vi "DSF.Engine.Transceiver Thread.Command.Transfer Group.vi"(8 "error in (no error)":errorcluster, 9 "Command":T1, 10 "Transfer Group":refnum<class "DSF.Engine.Transfer Group.lvclass">, 11 "Transceiver Thread in":refnum<class "DSF.Engine.Transceiver Thread.lvclass">) -> (0 "error out":errorcluster, 3 "Transceiver Thread out":refnum<class "DSF.Engine.Transceiver Thread.lvclass">)   [LabVIEW 2017, in "DSF.Engine.lvlib" / "DSF.Engine.Transceiver Thread.lvclass"]
uses:
  DSF.Engine.Transceiver Thread.lvclass
  Transfer/DSF.Engine.Transfer Group.lvclass
  Interface/DSF.Engine.Interface.Transceiver.Command.ctl
  Interface/DSF.Engine.Interface.Transceiver.Command Data.ctl
  Interface/DSF.Engine.Interface.Transceiver.Command Parameters.ctl
  DSF.Engine.Transceiver Thread.lvclass/DSF.Engine.Transceiver Thread.ctl
  Transfer/DSF.Engine.Transfer Group.lvclass/DSF.Engine.Transfer Group.ctl
  Timing/DSF.Engine.Timing.lvclass/DSF.Engine.Timing.ctl
  Interface/DSF.Engine.Interface.Transceiver.Write.Command.vi
  Interface/DSF.Engine.Interface.Transceiver.lvclass
  Timing/DSF.Engine.Timing.lvclass
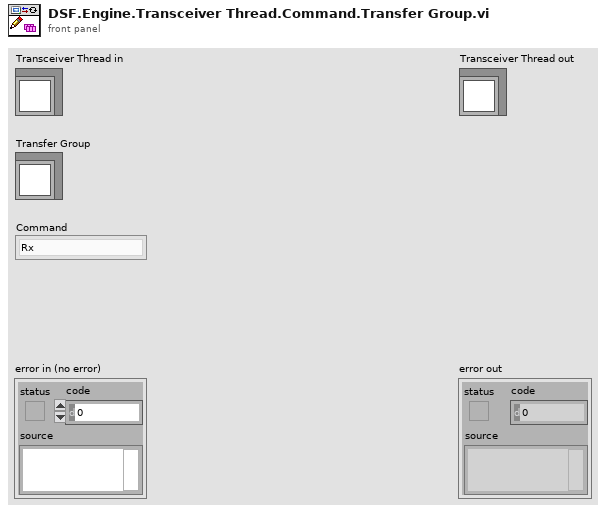
[diagram p1: front panel]
types:
  T1 = typedef "DSF.Engine.lvlib/DSF.Engine.Interface.Transceiver.lvclass/DSF.Engine.Interface.Transceiver.Command.ctl" = enum8{"Rx", "Tx", "Shutdown"}
  T2 = cluster{"Transfer Group ID":i32, "unused":i32, "Transfer Group iteration":u64}
  T3 = typedef "DSF.Engine.lvlib/DSF.Engine.Interface.Transceiver.lvclass/DSF.Engine.Interface.Transceiver.Command Parameters.ctl" = cluster{"arg1":u64, "arg2":u64}
  T4 = typedef "DSF.Engine.lvlib/DSF.Engine.Interface.Transceiver.lvclass/DSF.Engine.Interface.Transceiver.Command Data.ctl" = cluster{"Command":T1, "Command Parameters":T3}
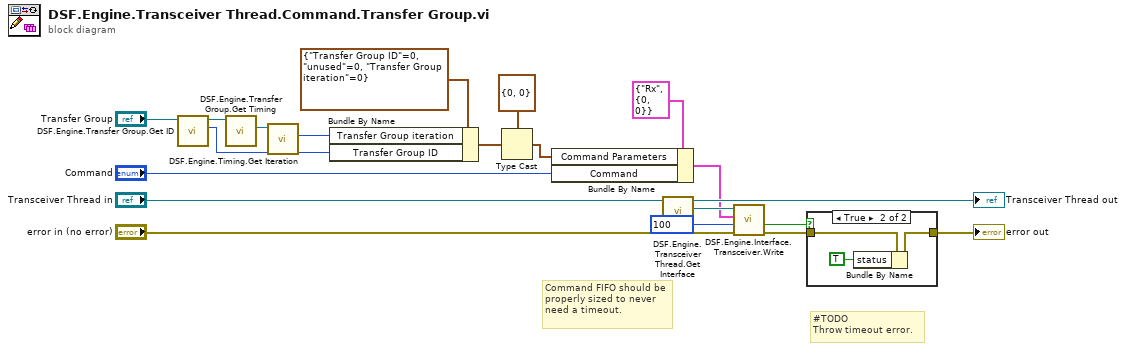
[diagram p0: block diagram]
diagram:
  # "Command FIFO should be properly sized to never need a timeout."
  # "#TODO\nThrow timeout error."
  n1 = call "DSF.Engine.Transfer Group.Get ID.vi"("Transfer Group in"="Transfer Group") -> ("id"=w9:i32, "Transfer Group out"=w8:refnum<class "DSF.Engine.Transfer Group.lvclass">)  [unwired: 9 in]
  n2 = call "DSF.Engine.Transfer Group.Get Timing.vi"("Transfer Group in"=w8) -> ("Timing"=w7:refnum<class "DSF.Engine.Timing.lvclass">)  [unwired: 9 in, 1 out]
  n3 = call "DSF.Engine.Timing.Get Iteration.vi"("Timing in"=w7) -> ("Iteration"=w6:u64)  [unwired: 9 in, 1 out]
  n4 = Bundle By Name(cluster=T2 {"Transfer Group ID"=0, "unused"=0, "Transfer Group iteration"=0}, "Transfer Group iteration"=w6, "Transfer Group ID"=w9) -> (w10:T2)
  n5 = Type Cast(type=T3 {"arg1"=0, "arg2"=0} ("Command Parameters"), x=w10) -> (*(type *) &x=w12:T3)
  n6 = Bundle By Name(cluster=T4 {"Command"=enum."Rx", "Command Parameters"={"arg1"=0, "arg2"=0}} ("command"), "Command Parameters"=w12, "Command"="Command") -> (w16:T4)
  n7 = call "DSF.Engine.Transceiver Thread.Get Interface.vi"("Transceiver Thread in"="Transceiver Thread in") -> ("Interface"=w18:refnum<class "DSF.Engine.Interface.Transceiver.lvclass">, "Transceiver Thread out"=→"Transceiver Thread out":refnum<class "DSF.Engine.Transceiver Thread.lvclass">)  [unwired: 9 in]
  n8 = call-poly "DSF.Engine.Interface.Transceiver.Write.vi"("error in (no error)"="error in (no error)", "timeout in ms (0)"=100, "command"=w16, "Transceiver Interface in"=w18) -> ("error out"=w4:errorcluster, "timed out?"=w5:bool)  [unwired: 5 in, 1 out]
  n9 = case shown="True" w5 {
    tunnel: w4 -> [w21 w24]
    tunnel: [w21 w23] -> w3
    frame False {
    }
    frame True {
      n10 = Bundle By Name(cluster=w24, "status"=TRUE) -> (w23:errorcluster)
    }
  }
  "error out" <- w3
